vi "Get_Frequency.vi"(8 "error in (no error)":errorcluster, 11 ".NET Reference in":refnum<k24>) -> (0 "error out":errorcluster, 2 "freq":dbl, 3 "Reference out":refnum<k24>)   [LabVIEW 2017]
uses:
  LV_IL_Sample/DLL/InstrumentDLL.dll
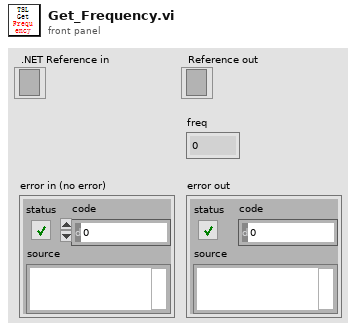
[diagram p1: front panel]
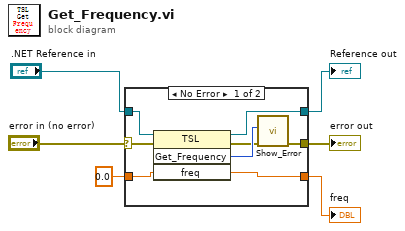
[diagram p0: block diagram]
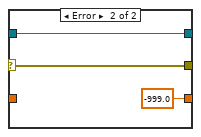
[diagram p2: hidden frame]
diagram:
  n1 = case shown="No Error" "error in (no error)" {
    selector: "error in (no error)" -> [w7 w17]
    tunnel: [w14 -999.0 ("freq")] -> w6
    tunnel: ".NET Reference in" -> [w13 w15]
    tunnel: [w12 w15] -> w4
    tunnel: [w8 w17] -> w3
    tunnel: 0.0 ("freq") -> [w11 _]
    frame No Error {
      n2 = invoke on="调用节点" class="TSL" method="Get_Frequency"(reference=w13, error in=w7, "freq"=w11) -> (reference out=w12:refnum<k24>, error out=w9:errorcluster, "Get_Frequency"=w10:i32, "freq"=w14:dbl)  [unwired: 1 in]
      n3 = call "Show_Error.vi"("error in (no error)"=w9, "Error"=w10) -> ("error out"=w8:errorcluster)  [unwired: 9 in]
    }
    frame Error {
    }
  }
  "freq" <- w6
  "Reference out" <- w4
  "error out" <- w3
